vi "Get Target Time Elapsed Event.vi"(8 "error in (no error)":errorcluster, 11 "Timed Door in":refnum<class "Timed Door.lvclass">) -> (0 "error out":errorcluster, 2 "Target Time Elapsed Event":refnum<user-event>, 3 "Timed Door out":refnum<class "Timed Door.lvclass">)   [LabVIEW 2018, in "Timed Door.lvclass"]
uses:
  Timed Door.lvclass
  Timed Door.lvclass/Timed Door.ctl
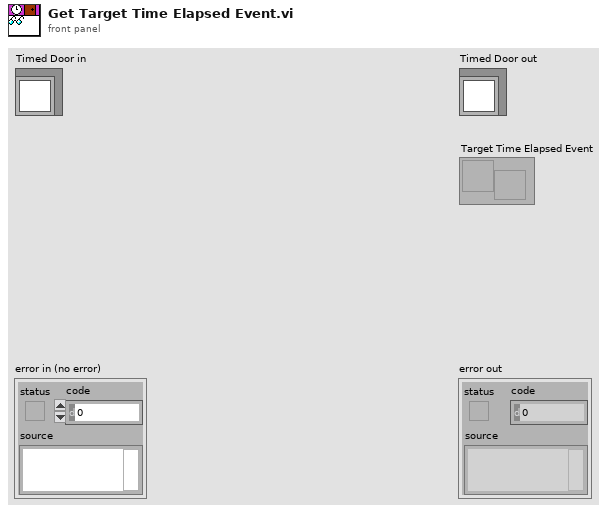
[diagram p1: front panel]
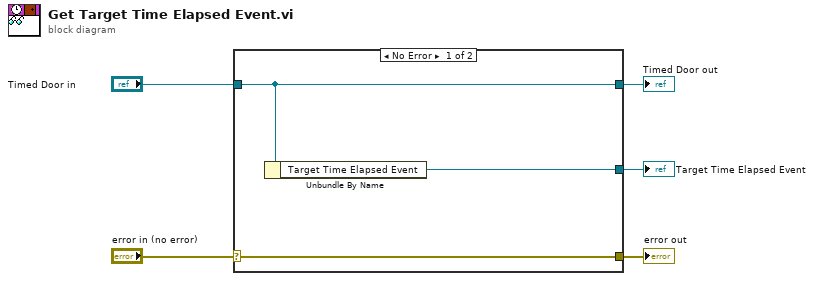
[diagram p0: block diagram]
diagram:
  n1 = case shown="No Error" "error in (no error)" {
    selector: "error in (no error)" -> [w8 w9]
    tunnel: [w8 w9] -> w4
    tunnel: [w7 w10] -> w2
    tunnel: "Timed Door in" -> [w7 w10]
    tunnel: [w6 _] -> w1
    frame No Error {
      n2 = Unbundle By Name(w7) -> ("Target Time Elapsed Event"=w6:refnum<user-event>)
    }
    frame Error {
    }
  }
  "error out" <- w4
  "Timed Door out" <- w2
  "Target Time Elapsed Event" <- w1
